vi "Write TCS Infos.vi"(8 "error in (no error)":errorcluster, 10 "TCS Infos":T1, 11 "TCS in":refnum<class "TCS.lvclass">) -> (0 "error out":errorcluster, 3 "TCS out":refnum<class "TCS.lvclass">)   [LabVIEW 2018, in "TCS.lvclass"]
uses:
  TCS.lvclass
  TCS.lvclass/TCS.ctl
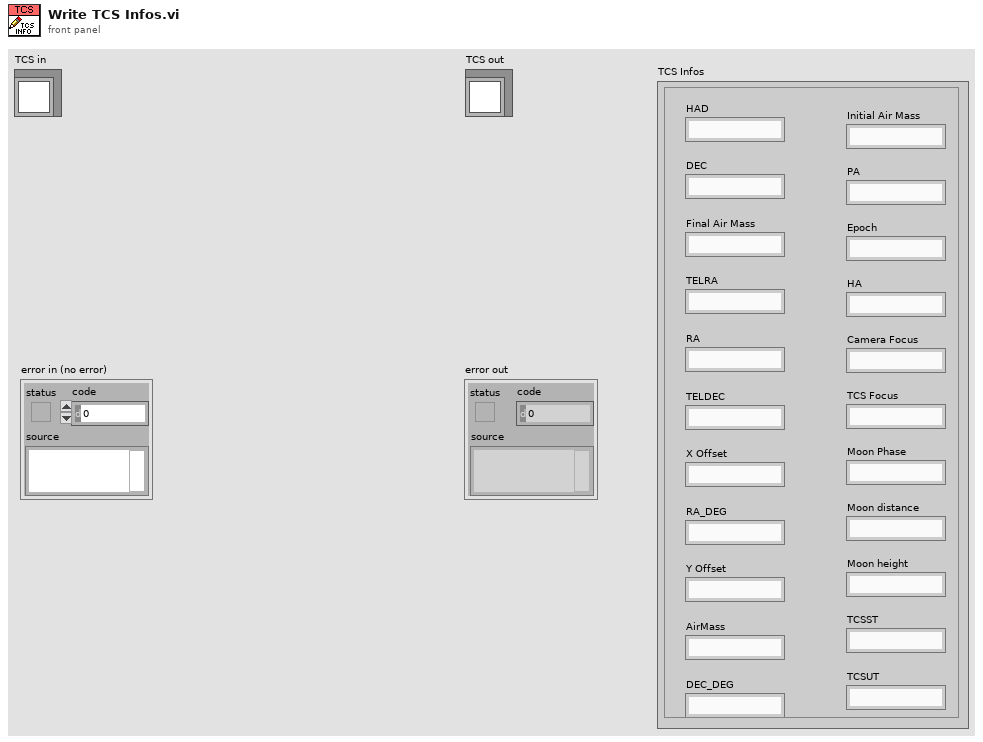
[diagram p1: front panel]
types:
  T1 = cluster{"RA":string, "DEC":string, "TELRA":string, "TELDEC":string, "RA_DEG":string, "DEC_DEG":string, "Epoch":string, "AirMass":string, "Initial Air Mass":string, "HA":string, "HAD":string, "Final Air Mass":string, "X Offset":string, "Y Offset":string, "PA":string, "Camera Focus":string, "TCS Focus":string, "Moon distance":string, "Moon height":string, "Moon Phase":string, "TCSST":string, "TCSUT":string}
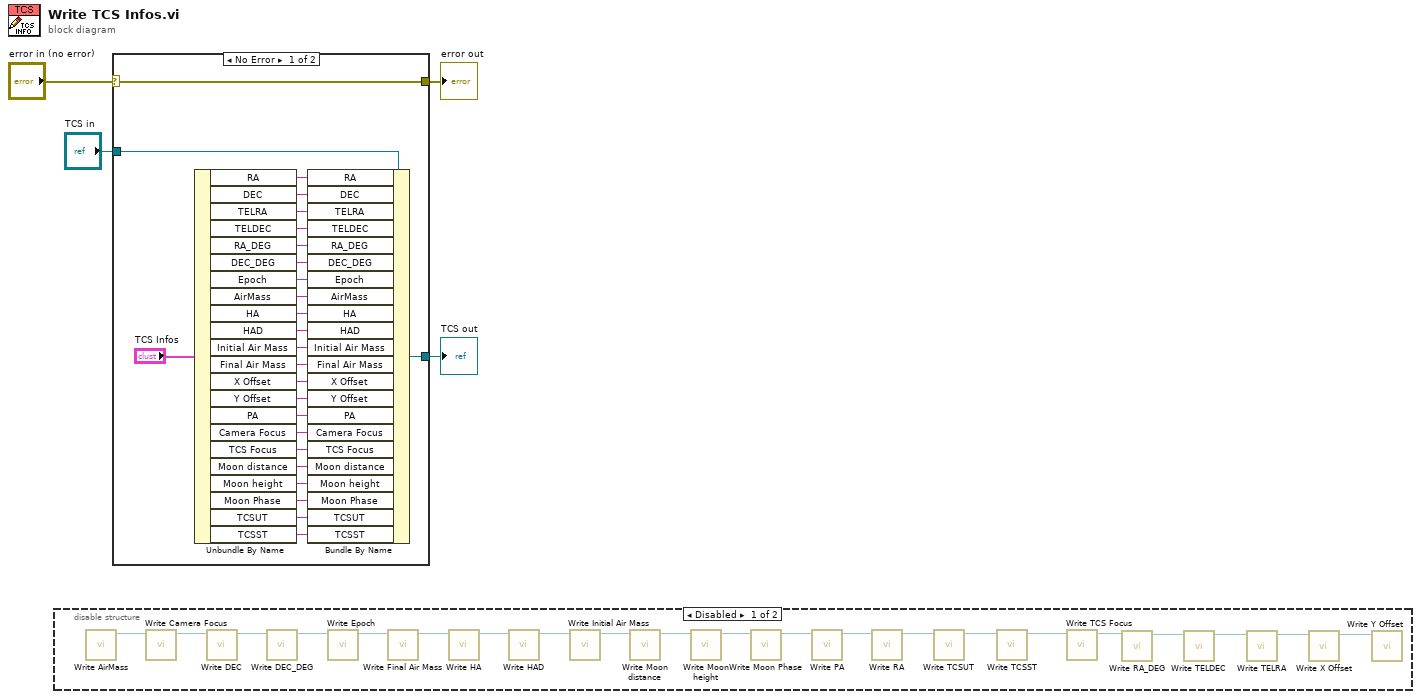
[diagram p0: block diagram]
diagram:
  n1 = disable-structure shown="Disabled" {
    frame Disabled {
      n2 = call "Write AirMass.vi"() -> ("TCS out"=w5:refnum<class "TCS.lvclass">)  [unwired: 10 in, 1 out]
      n3 = call "Write Camera Focus.vi"("TCS in"=w5) -> ("TCS out"=w6:refnum<class "TCS.lvclass">)  [unwired: 9 in, 1 out]
      n4 = call "Write DEC.vi"("TCS in"=w6) -> ("TCS out"=w7:refnum<class "TCS.lvclass">)  [unwired: 9 in, 1 out]
      n5 = call "Write DEC_DEG.vi"("TCS in"=w7) -> ("TCS out"=w8:refnum<class "TCS.lvclass">)  [unwired: 9 in, 1 out]
      n6 = call "Write Epoch.vi"("TCS in"=w8) -> ("TCS out"=w9:refnum<class "TCS.lvclass">)  [unwired: 9 in, 1 out]
      n7 = call "Write Final Air Mass.vi"("TCS in"=w9) -> ("TCS out"=w10:refnum<class "TCS.lvclass">)  [unwired: 9 in, 1 out]
      n8 = call "Write HA.vi"("TCS in"=w10) -> ("TCS out"=w11:refnum<class "TCS.lvclass">)  [unwired: 9 in, 1 out]
      n9 = call "Write HAD.vi"("TCS in"=w11) -> ("TCS out"=w12:refnum<class "TCS.lvclass">)  [unwired: 9 in, 1 out]
      n10 = call "Write Initial Air Mass.vi"("TCS in"=w12) -> ("TCS out"=w13:refnum<class "TCS.lvclass">)  [unwired: 9 in, 1 out]
      n11 = call "Write Moon distance.vi"("TCS in"=w13) -> ("TCS out"=w14:refnum<class "TCS.lvclass">)  [unwired: 9 in, 1 out]
      n12 = call "Write Moon height .vi"("TCS in"=w14) -> ("TCS out"=w15:refnum<class "TCS.lvclass">)  [unwired: 9 in, 1 out]
      n13 = call "Write Moon Phase.vi"("TCS in"=w15) -> ("TCS out"=w16:refnum<class "TCS.lvclass">)  [unwired: 9 in, 1 out]
      n14 = call "Write PA.vi"("TCS in"=w16) -> ("TCS out"=w17:refnum<class "TCS.lvclass">)  [unwired: 9 in, 1 out]
      n15 = call "Write RA.vi"("TCS in"=w17) -> ("TCS out"=w18:refnum<class "TCS.lvclass">)  [unwired: 9 in, 1 out]
      n16 = call "Write TCSUT.vi"("TCS in"=w18) -> ("TCS out"=w19:refnum<class "TCS.lvclass">)  [unwired: 9 in, 1 out]
      n17 = call "Write TCSST.vi"("TCS in"=w19) -> ("TCS out"=w20:refnum<class "TCS.lvclass">)  [unwired: 9 in, 1 out]
      n18 = call "Write TCS Focus.vi"("TCS in"=w20) -> ("TCS out"=w21:refnum<class "TCS.lvclass">)  [unwired: 9 in, 1 out]
      n19 = call "Write RA_DEG.vi"("TCS in"=w21) -> ("TCS out"=w22:refnum<class "TCS.lvclass">)  [unwired: 9 in, 1 out]
      n20 = call "Write TELDEC.vi"("TCS in"=w22) -> ("TCS out"=w23:refnum<class "TCS.lvclass">)  [unwired: 9 in, 1 out]
      n21 = call "Write TELRA.vi"("TCS in"=w23) -> ("TCS out"=w24:refnum<class "TCS.lvclass">)  [unwired: 9 in, 1 out]
      n22 = call "Write X Offset.vi"("TCS in"=w24) -> ("TCS out"=w25:refnum<class "TCS.lvclass">)  [unwired: 9 in, 1 out]
      n23 = call "Write Y Offset.vi"("TCS in"=w25) -> ()  [unwired: 9 in, 2 out]
    }
    frame Enabled {
    }
  }
  n24 = case shown="No Error" "error in (no error)" {
    selector: "error in (no error)" -> [w51 w53]
    tunnel: [w51 w53] -> w3
    tunnel: [w49 w52] -> w1
    tunnel: "TCS in" -> [w50 w52]
    frame No Error {
      n25 = Unbundle By Name("TCS Infos") -> ("RA"=w47:string, "DEC"=w46:string, "TELRA"=w45:string, "TELDEC"=w44:string, "RA_DEG"=w43:string, "DEC_DEG"=w42:string, "Epoch"=w41:string, "AirMass"=w40:string, "HA"=w39:string, "HAD"=w38:string, "Initial Air Mass"=w37:string, "Final Air Mass"=w36:string, "X Offset"=w35:string, "Y Offset"=w34:string, "PA"=w33:string, "Camera Focus"=w32:string, "TCS Focus"=w31:string, "Moon distance"=w30:string, "Moon height"=w29:string, "Moon Phase"=w28:string, "TCSUT"=w27:string, "TCSST"=w26:string)
      n26 = Bundle By Name(cluster=w50, "RA"=w47, "DEC"=w46, "TELRA"=w45, "TELDEC"=w44, "RA_DEG"=w43, "DEC_DEG"=w42, "Epoch"=w41, "AirMass"=w40, "HA"=w39, "HAD"=w38, "Initial Air Mass"=w37, "Final Air Mass"=w36, "X Offset"=w35, "Y Offset"=w34, "PA"=w33, "Camera Focus"=w32, "TCS Focus"=w31, "Moon distance"=w30, "Moon height"=w29, "Moon Phase"=w28, "TCSUT"=w27, "TCSST"=w26) -> (w49:refnum<class "TCS.lvclass">)
    }
    frame Error {
    }
  }
  "error out" <- w3
  "TCS out" <- w1
